vi "Finalize.vi"(8 "Error in":errorcluster, 10 "Msg Output":refnum<class "Msg Output.lvclass">, 11 "Base Actor in":refnum<class "Base Actor.lvclass">) -> (0 "Error out":errorcluster, 3 "Base Actor out":refnum<class "Base Actor.lvclass">)   [LabVIEW 2020, in "jettl.lvlib" / "Base jettl Actor.lvlib" / "Base Actor.lvlib" / "Base Actor.lvclass"]
uses:
  Base Actor.lvclass
  Msg Output/Msg Output.lvclass
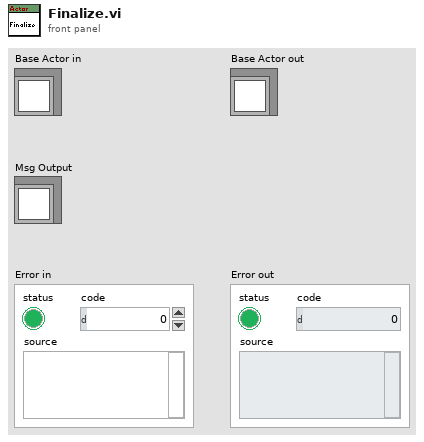
[diagram p1: front panel]
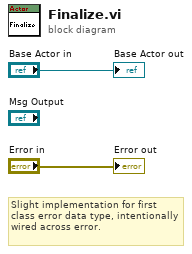
[diagram p0: block diagram]
diagram:
  # "Slight implementation for first class error data type, intentionally wired across error."
  "Base Actor out" <- "Base Actor in"
  "Error out" <- "Error in"
